vi "DISP_WIND_TRAC_Y_SCAL_RLEV.vi"(0 "VISA IN":refnum<visa-resource-name>, 1 "Trace":i32=1, 2 "Ref Level":i32=1, 5 "error in":errorcluster, 7 "Window":i32=1) -> (14 "VISA Out":refnum<visa-resource-name>, 19 "error out":errorcluster)   [LabVIEW 2018, in "PNA-X.lvlib"]
doc: "DISPlay:WINDow<wnum>:TRACe<tnum>:Y[:SCALe]:RLEVel <num> \n1599\n\n(Read-Write) Sets the Y axis Reference Level of the specified trace in the specified window. \nParameters \n<wnum> Any existing window number. If unspecified, value is set to 1. \n<tnum> Any existing trace number; if unspecified, value is set to 1 \n<num> Reference level value. The range of acceptable values is dependent on format \nand domain. \nNote: This command will accept MIN or MAX instead of a numeric parameter. \nSee SCPI Syntax for more information. \nExamples DISP:WIND:TRAC:Y:RLEV 0 \ndisplay:window2:trace2:y:scale:rlevel minimum \nQuery Syntax DISPlay:WINDow<wnum>:TRACe<tnum>:Y[:SCALe]:RLEVel? \nReturn Type Numeric \nDefault NA"
uses:
  PNA-X.lvlib
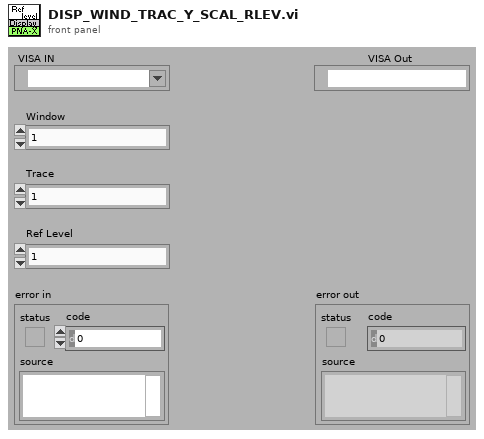
[diagram p1: front panel]
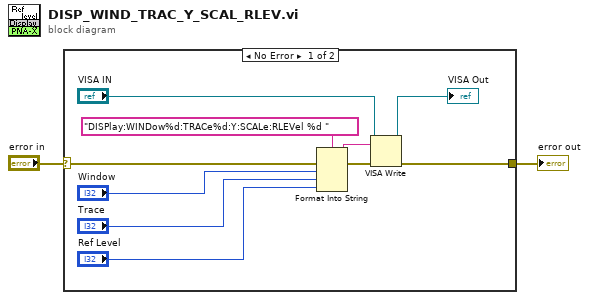
[diagram p0: block diagram]
diagram:
  n1 = case shown="No Error" "error in" {
    selector: "error in" -> [w12 w13]
    tunnel: [w7 w13] -> w1
    frame No Error {
      n2 = Format Into String(format string="DISPlay:WINDow%d:TRACe%d:Y:SCALe:RLEVel %d " ("Cmdline"), error in=w12, "Window", "Trace", "Ref Level") -> (resulting string=w10:string, error out=w11:errorcluster)  [unwired: 1 in]
      n3 = VISA Write(VISA resource name="VISA IN", write buffer=w10, error in (no error)=w11) -> (VISA resource name out=→"VISA Out":refnum<visa-resource-name>, error out=w7:errorcluster)  [unwired: 1 out]
    }
    frame Error {
    }
  }
  "error out" <- w1
